vi "Error Function.vi"(3 "x":dbl format="%.2f") -> (1 "erf(x)":dbl format="%.2f")   [LabVIEW 2020, in "NI_Gmath.lvlib"]
doc: "Computes the error function."
uses:
  NI_Gmath.lvlib
  <resource>/lvanlys.dll
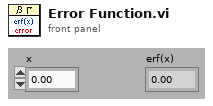
[diagram p1: front panel]
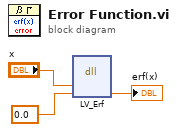
[diagram p0: block diagram]
diagram:
  n1 = dll-call lib="C:/Program Files (x86)/National Instruments/LabVIEW 2020/resource/lvanlys.*" fn="LV_Erf"("x"="x", "Erf(x)"=0.0 ("Erf")) -> ("Erf(x)"=→"erf(x)":dbl)  [unwired: 5 in, 2 out]
